vi "User_Database_Query.vi"(7 "Read?":bool, 8 "error in (no error)":errorcluster caption="Error In", 10 "SQL query":string, 11 "SQLite Connection in":refnum<class "Connection.lvclass">) -> (0 "error out":errorcluster caption="Error Out", 2 "Data":string[][](array[string]), 3 "SQLite Connection":refnum<class "Connection.lvclass">)   [LabVIEW 2020]
uses:
  <vilib>/drjdpowell/SQLite Library/SQL Connection/Connection.lvclass
  <vilib>/drjdpowell/SQLite Library/SQL Connection/Execute SQL.vi
  <vilib>/drjdpowell/SQLite Library/SQLite.lvlib
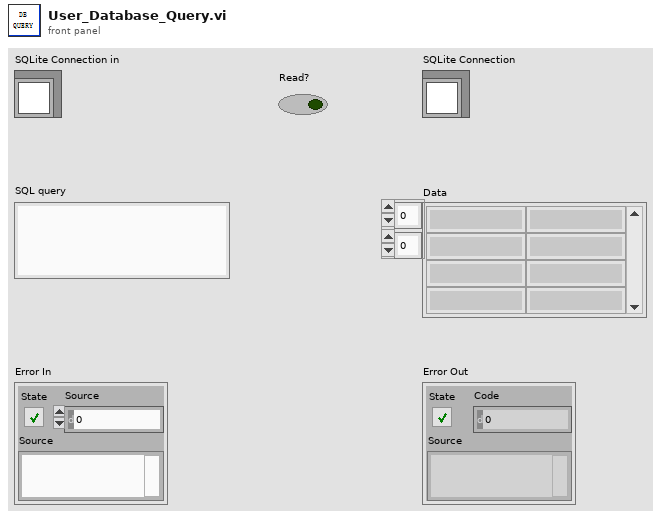
[diagram p1: front panel]
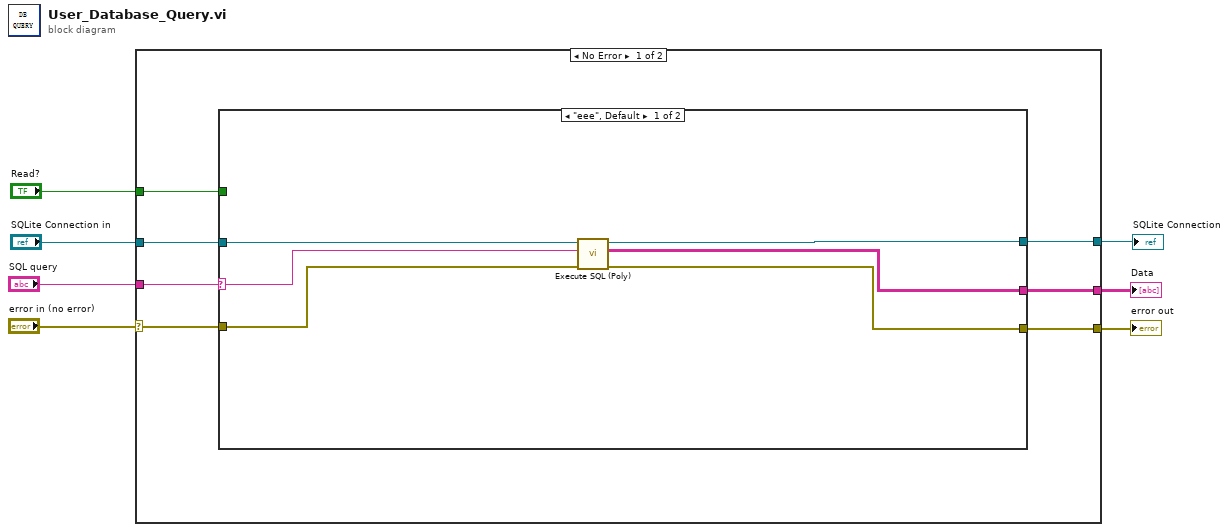
[diagram p0: block diagram]
diagram:
  n1 = case shown="No Error" "error in (no error)" {
    selector: "error in (no error)" -> [w14 w24]
    tunnel: [w13 w24] -> w4
    tunnel: "SQL query" -> [w12 _]
    tunnel: [w11 _] -> w6
    tunnel: "Read?" -> [w10 _]
    tunnel: "SQLite Connection in" -> [w9 w23]
    tunnel: [w8 w23] -> w1
    frame No Error {
      n2 = case shown="\"eee\", Default" w12 {
        selector: w12 -> [w19 _]
        tunnel: w14 -> [w18 w22]
        tunnel: [w17 w22] -> w13
        tunnel: [w20 _] -> w11
        tunnel: w10 -> [_ _]
        tunnel: w9 -> [w16 w21]
        tunnel: [w15 w21] -> w8
        frame "eee", Default {
          n3 = call-poly <vilib>:"Execute SQL (Poly).vi"("error in (no error)"=w18, "SQL"=w19, "SQLite Connection in"=w16) -> ("error out"=w17:errorcluster, "Result Set"=w20:string[][], "SQLite Connection"=w15:refnum<class "Connection.lvclass">)  [unwired: 5 in, 1 out]
        }
        frame "" {
        }
      }
    }
    frame Error {
    }
  }
  "error out" <- w4
  "Data" <- w6
  "SQLite Connection" <- w1
